vi "PH_gentec_P-Link.set Wavelength.vi"(0 "i ref in":refnum<vi>, 2 "VISA resource in":refnum<visa-resource-name>, 5 "error in":errorcluster) -> (11 "Timeout":bool, 13 "Data read":string[](array[string]), 14 "i ref out":refnum<vi>, 16 "VISA resource out":refnum<visa-resource-name>, 17 "Error":bool, 18 "Failure":bool, 19 "error out":errorcluster)   [LabVIEW 2014, in "PH_gentec_P-Link.lvlib"]
doc: "This VI writes wanted Settings to the Device and checks the result."
uses:
  PH_gentec_P-Link.lvlib
  PH_Basics/PH_Powermeter_BaseClass/PH_Powermeter_BaseClass.lvlib
  instr.lib/Gentec-P-Link/gentec-P-Link - Driver.lvlib
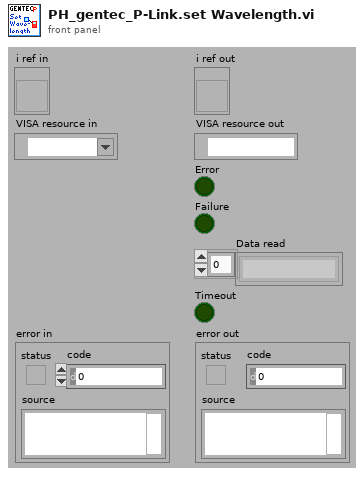
[diagram p1: front panel]
types:
  T1 = typedef "PH_Powermeter_BaseClass.lvlib/PH_Powermeter_BaseClass.i attribute.ctl" = cluster{"GUI References":T2, "Connection":T3, "Head Attributes":T5, "VISA resource":refnum<visa-resource-name>, "Energy":T6, "Service ID Energy":i32, "Wanted Settings":T7, "Current Settings":T7}
  T2 = typedef "PH_Powermeter_BaseClass.lvlib/PH_Powermeter_BaseClass.GUI Refs.ctl" = cluster{"Head Attributes":refnum<vi>, "Energy":refnum<vi>, "Connection":refnum<vi>, "VISA Resource":refnum<vi>, "Scaling Factor":refnum<vi>, "Range":refnum<vi>, "Wavelength":refnum<vi>, "Trigger Level":refnum<vi>, "Wanted Settings":refnum<vi>, "Current Settings":refnum<vi>}
  T3 = typedef "PH_Powermeter_BaseClass.lvlib/PH_Powermeter_BaseClass.Connection.ctl" = cluster{"failed checks":i8, "Timeout":bool, "Data read":string, "Failure":bool, "Error":bool, "State":T4}
  T4 = typedef "PH_Powermeter_BaseClass.lvlib/PH_Powermeter_BaseClass.State.ctl" = enum32{"off", "operating", "opened", "checked", "connected", "Sets to change", "running"}
  T5 = typedef "PH_Powermeter_BaseClass.lvlib/PH_Powermeter_BaseClass.Head Attributes.ctl" = cluster{"Instrument Type":string, "Head Version":string, "Head Name":string, "Serial Number":string, "Firmware":string, "Sensor Type":string, "MinimumRange":u32, "Maximum Range":u32, "Min Wavelength":i32, "Max Wavelength":i32}
  T6 = typedef "PH_Powermeter_BaseClass.lvlib/PH_Powermeter_BaseClass.Energy.ctl" = cluster{"current Value":dbl, "unscaled":dbl, "Scaling Factor":dbl}
  T7 = typedef "PH_Powermeter_BaseClass.lvlib/PH_gentec_BaseClass.Head Settings.ctl" = cluster{"Trigger Level":dbl, "Wavelength":u32, "Range":u32}
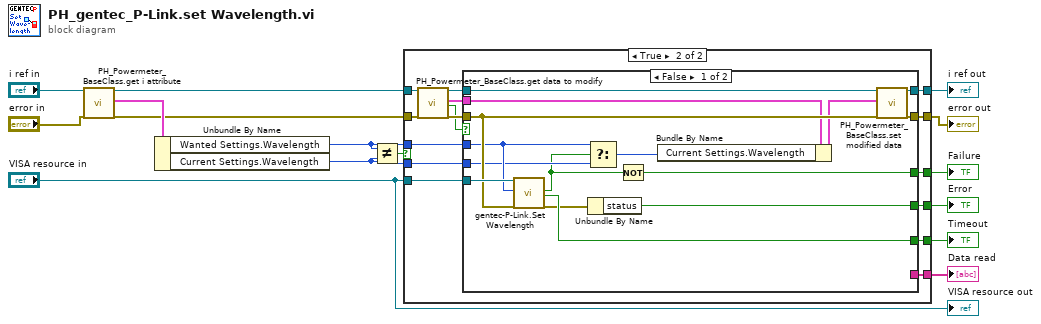
[diagram p0: block diagram]
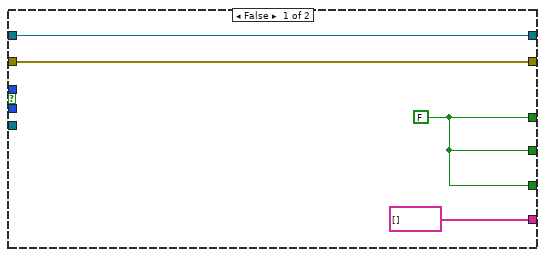
[diagram p2: hidden frame]
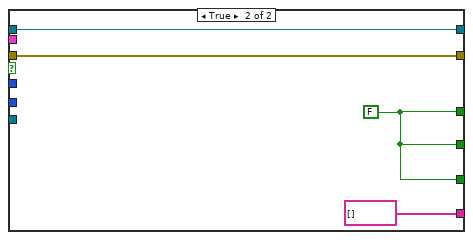
[diagram p3: hidden frame]
diagram:
  n1 = call "PH_Powermeter_BaseClass.get i attribute.vi"("i ref in"="i ref in", "error in (no error)"="error in") -> ("i ref out"=w9:refnum<vi>, "i attribute"=w12:T1, "error out"=w11:errorcluster)  [unwired: 15 in]
  n2 = Unbundle By Name(w12) -> ("Wanted Settings.Wavelength"=w13:u32, "Current Settings.Wavelength"=w1:u32)
  n3 = Not Equal?(x=w13, y=w1) -> (x != y?=w2:bool)
  n4 = case shown="True" w2 {
    tunnel: [w16 w34] -> w15
    tunnel: [w17 w33] -> w14
    tunnel: w13 -> [_ w32]
    tunnel: w11 -> [w16 w27]
    tunnel: w9 -> [w17 w26]
    tunnel: "VISA resource in" -> [_ w25]
    tunnel: [w19 w24] -> w6
    tunnel: [w19 w23] -> w5
    tunnel: [w19 w22] -> w4
    tunnel: [string[] [] w20] -> w3
    tunnel: w1 -> [_ w21]
    frame False {
      w19 = FALSE
    }
    frame True {
      n5 = call "PH_Powermeter_BaseClass.get data to modify.vi"("i ref in"=w26, "error in (no error)"=w27) -> ("i ref out"=w30:refnum<vi>, "i attribute"=w29:T1, "timed out"=w28:bool, "error out"=w31:errorcluster)  [unwired: 14 in]
      n6 = case shown="False" w28 {
        tunnel: w25 -> [w48 _]
        tunnel: [w45 w53] -> w33
        tunnel: [w44 w52] -> w34
        tunnel: w31 -> [w47 w52]
        tunnel: w30 -> [w49 w53]
        tunnel: w29 -> [w46 _]
        tunnel: w32 -> [w39 _]
        tunnel: [w42 w51] -> w24
        tunnel: [w35 w51] -> w23
        tunnel: [w41 w51] -> w22
        tunnel: w21 -> [w37 _]
        tunnel: [_ string[] []] -> w20
        frame False {
          n7 = call "gentec-P-Link.Set Wavelength.vi"("VISA resource name"=w48, "Wavelength (nm)"=w39, "error in (no error)"=w47) -> ("Sucess?"=w36:bool, "TimeOut?"=w41:bool, "error out"=w38:errorcluster)  [unwired: 13 in, 1 out]
          n8 = Select(t=w39, s=w36, f=w37) -> (s? t:f=w40:u32)
          n9 = Unbundle By Name(w38) -> ("status"=w42:bool)
          n10 = Not(x=w36) -> (.not. x?=w35:bool)
          n11 = Bundle By Name(cluster=w46, "Current Settings.Wavelength"=w40) -> (w43:T1)
          n12 = call "PH_Powermeter_BaseClass.set modified data.vi"("i ref in"=w49, "i attribute"=w43, "error in (no error)"=w47) -> ("i ref out"=w45:refnum<vi>, "error out"=w44:errorcluster)  [unwired: 15 in]
        }
        frame True {
          w51 = FALSE
        }
      }
    }
  }
  "error out" <- w15
  "i ref out" <- w14
  "Error" <- w6
  "Failure" <- w5
  "Timeout" <- w4
  "Data read" <- w3
  "VISA resource out" <- "VISA resource in"
